vi "atividade 1 nauka.vi"() -> ()   [LabVIEW 2024]
panel:
  out "Indicator 1":bool
  out "Slide":dbl(slide) scale=0.0..100.0
  in  "Boolean 2":bool
  out "Boolean":bool=TRUE
  out "String":string="essa e uma string"
  in  "VALOR N":dbl
  in  "ARRAY 2-1":dbl
  in  "ARRAY 2-0":dbl
  in  "ARRAY 1-1":dbl
  in  "ARRAY 1-0":dbl
  out "Numeric":i32
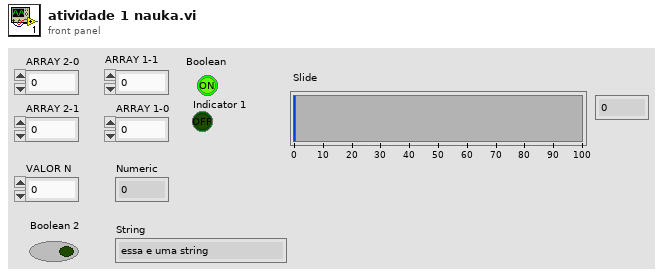
[diagram p1: front panel]
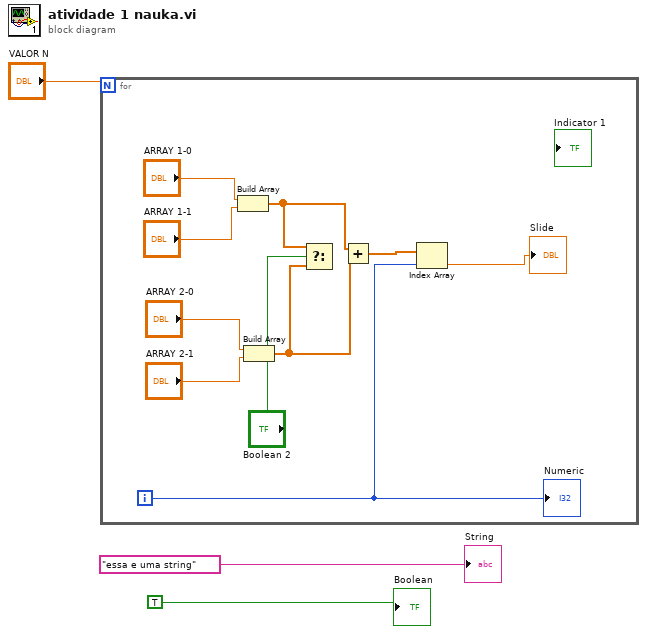
[diagram p0: block diagram]
diagram:
  n1 = for {
    N: "VALOR N" -> [_]
    i -> [w8]
    n2 = Build Array("ARRAY 1-0", "ARRAY 1-1") -> (w7:dbl[])
    n3 = Build Array("ARRAY 2-0", "ARRAY 2-1") -> (w6:dbl[])
    n4 = Select(t=w7, s="Boolean 2", f=w6) -> ()  [unwired: 1 out]
    n5 = Add(x=w7, y=w6) -> (x+y=w9:dbl[])
    n6 = Index Array(array=w9, index=w8) -> (element=→"Slide":dbl)
    "Numeric" <- w8
  }
  "String" <- "essa e uma string"
  "Boolean" <- TRUE
